vi "Read % Dead Zone Y-Axis.vi"(8 "error in (no error)":errorcluster, 11 "Joystick Guidance in":refnum<class "Joystick Guidance.lvclass">) -> (0 "error out":errorcluster, 2 "% Dead Zone Y-Axis":dbl, 3 "Joystick Guidance out":refnum<class "Joystick Guidance.lvclass">)   [LabVIEW 2011, in "Guidance Library.lvlib" / "Joystick Guidance.lvclass"]
uses:
  Joystick Guidance.lvclass
  Joystick Guidance.lvclass/Joystick Guidance.ctl
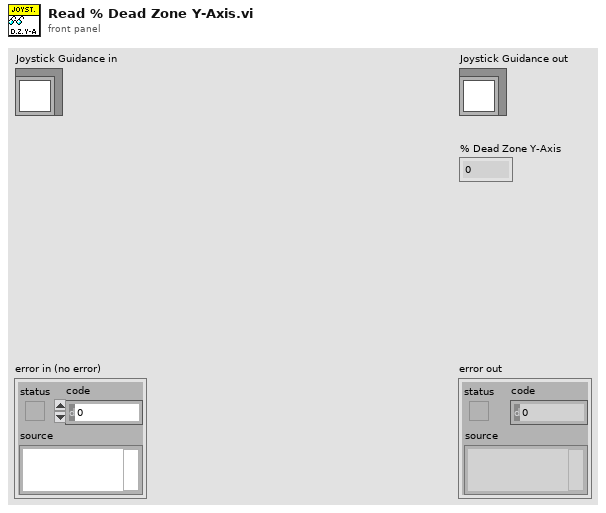
[diagram p1: front panel]
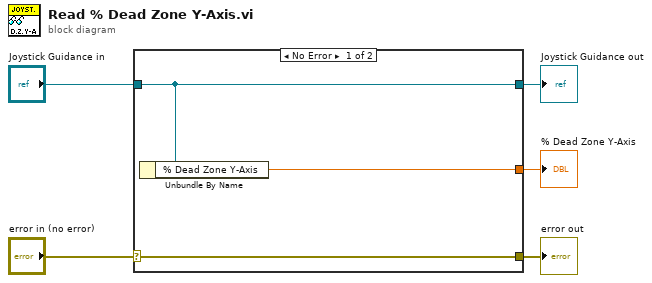
[diagram p0: block diagram]
diagram:
  n1 = case shown="No Error" "error in (no error)" {
    selector: "error in (no error)" -> [w8 w9]
    tunnel: [w8 w9] -> w4
    tunnel: [w7 w10] -> w2
    tunnel: "Joystick Guidance in" -> [w7 w10]
    tunnel: [w6 _] -> w1
    frame No Error {
      n2 = Unbundle By Name(w7) -> ("% Dead Zone Y-Axis"=w6:dbl)
    }
    frame Error {
    }
  }
  "error out" <- w4
  "Joystick Guidance out" <- w2
  "% Dead Zone Y-Axis" <- w1
